vi "sortLinesAndVolumes.vi"(8 "error in (no error)":errorcluster, 9 "new volumes":T4(array[cluster]), 10 "Array of lines":T3(array[cluster]), 11 "assembler status":T2) -> (0 "error out":errorcluster, 1 "volumes to assemble":T1(array[cluster]), 2 "leftover lines":T3(array[cluster]), 3 "assembler status out":T2, 4 "num volume ends":i16, 5 "lines lost":i32)   [LabVIEW 2010]
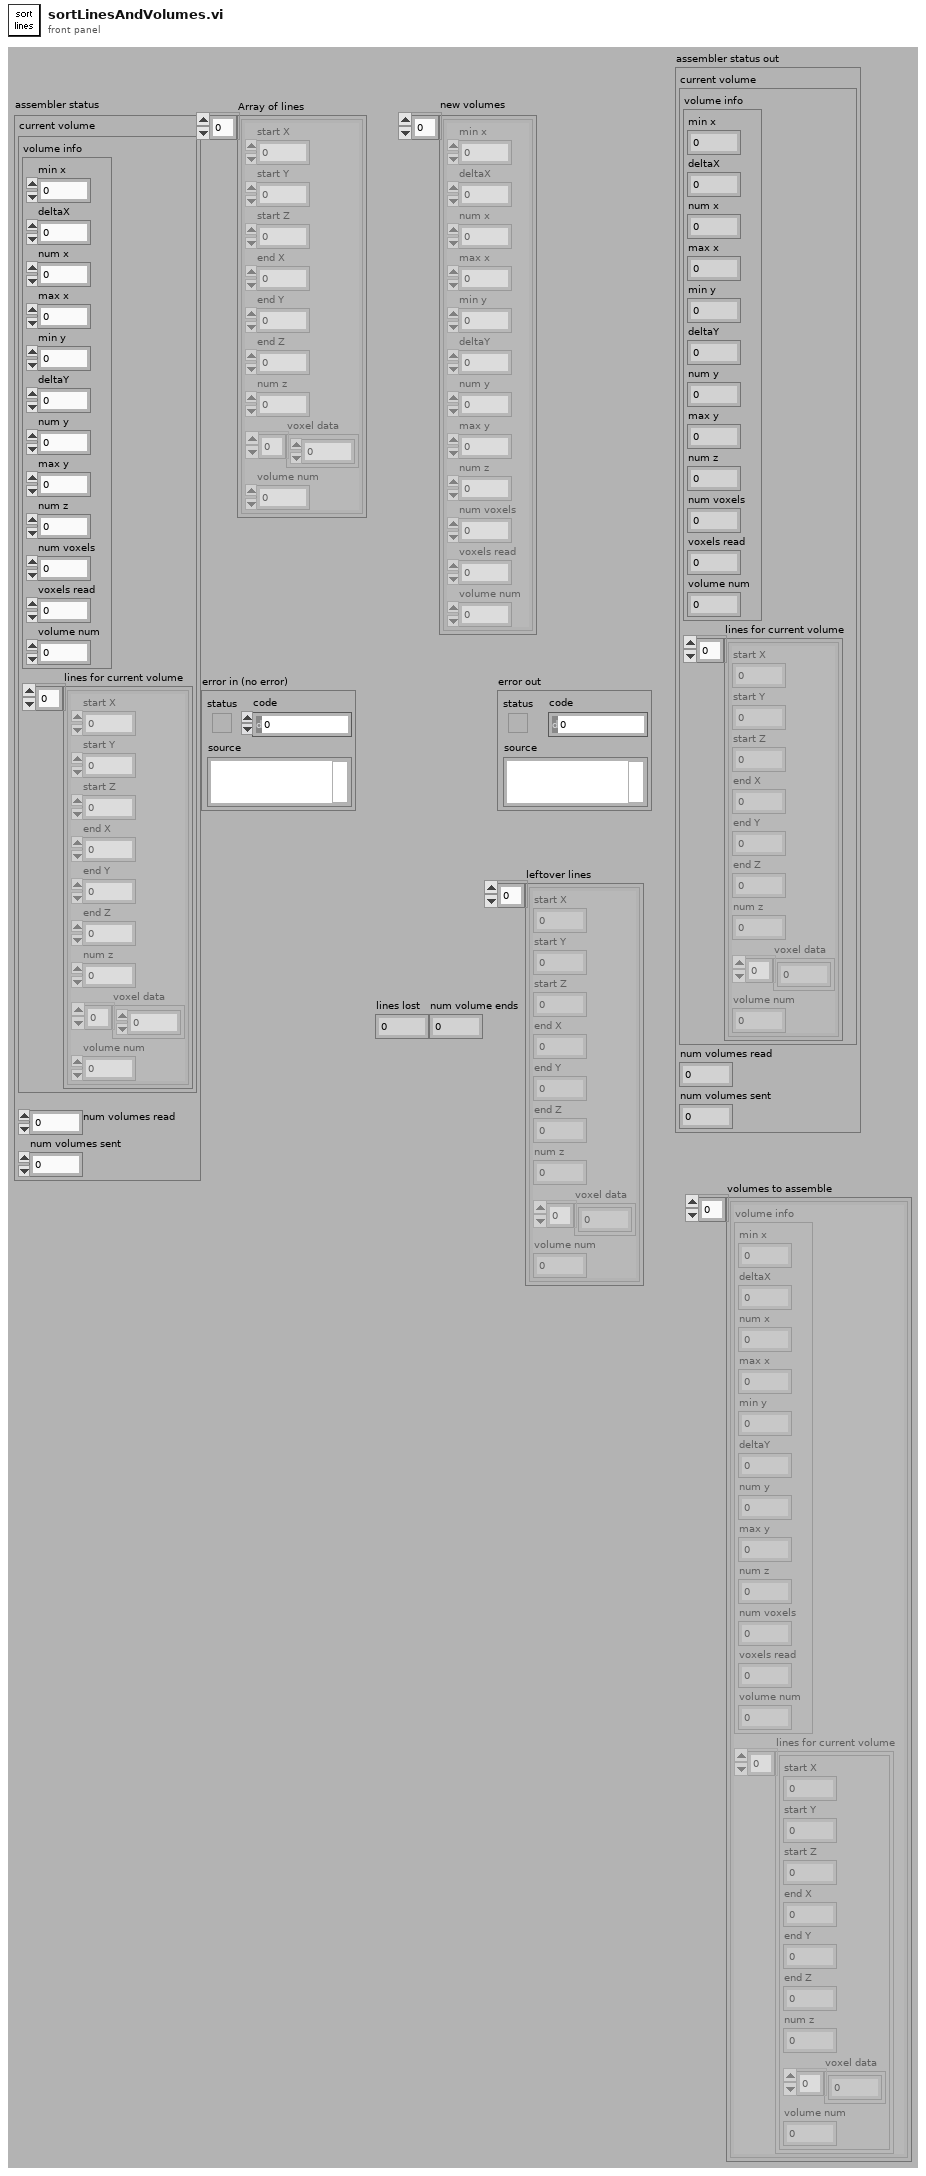
[diagram p1: front panel]
types:
  T1 = cluster{"volume info":cluster{"min x":i16, "deltaX":dbl, "num x":u32, "max x":i16, "min y":i16, "deltaY":dbl, "num y":u32, "max y":i16, "num z":u32, "num voxels":u32, "voxels read":u32, "volume num":u32}, "lines for current volume":cluster{"start X":i16, "start Y":i16, "start Z":i16, "end X":i16, "end Y":i16, "end Z":i16, "num z":u8, "voxel data":u32[], "volume num":u32}[]}[]
  T2 = cluster{"current volume":cluster{"volume info":cluster{"min x":i16, "deltaX":dbl, "num x":u32, "max x":i16, "min y":i16, "deltaY":dbl, "num y":u32, "max y":i16, "num z":u32, "num voxels":u32, "voxels read":u32, "volume num":u32}, "lines for current volume":cluster{"start X":i16, "start Y":i16, "start Z":i16, "end X":i16, "end Y":i16, "end Z":i16, "num z":u8, "voxel data":u32[], "volume num":u32}[]}, "num volumes read":u32, "num volumes sent":u32}
  T3 = cluster{"start X":i16, "start Y":i16, "start Z":i16, "end X":i16, "end Y":i16, "end Z":i16, "num z":u8, "voxel data":u32[], "volume num":u32}[]
  T4 = cluster{"min x":i16, "deltaX":dbl, "num x":u32, "max x":i16, "min y":i16, "deltaY":dbl, "num y":u32, "max y":i16, "num z":u32, "num voxels":u32, "voxels read":u32, "volume num":u32}[]
  T5 = cluster{"volume info":cluster{"min x":i16, "deltaX":dbl, "num x":u32, "max x":i16, "min y":i16, "deltaY":dbl, "num y":u32, "max y":i16, "num z":u32, "num voxels":u32, "voxels read":u32, "volume num":u32}, "lines for current volume":cluster{"start X":i16, "start Y":i16, "start Z":i16, "end X":i16, "end Y":i16, "end Z":i16, "num z":u8, "voxel data":u32[], "volume num":u32}[]}
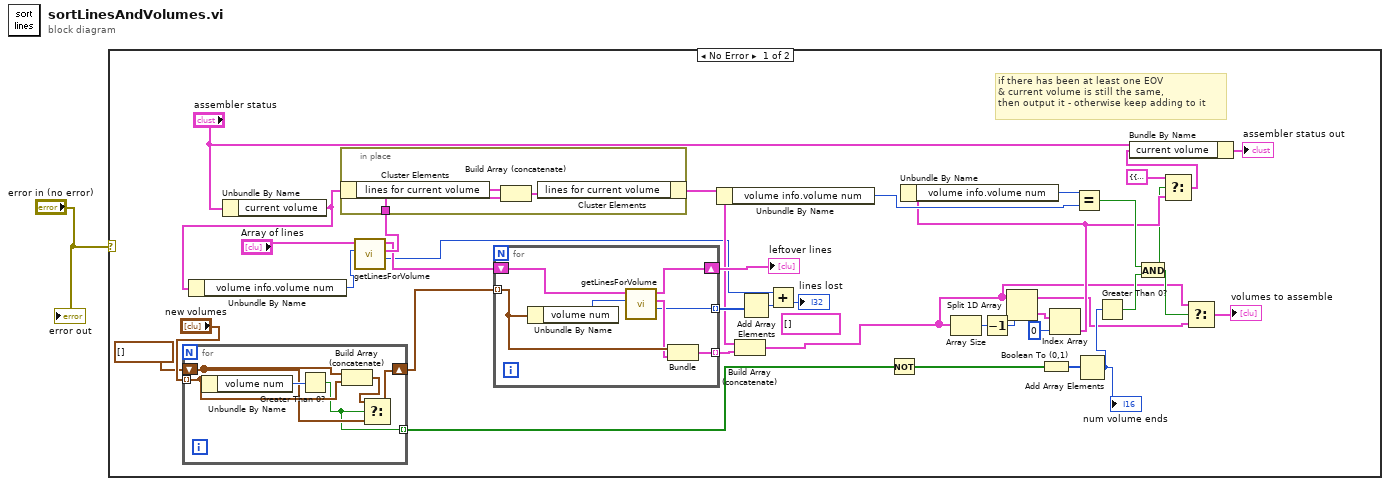
[diagram p0: block diagram]
diagram:
  n1 = case shown="No Error" "error in (no error)" {
    frame No Error {
      (unwired) T1 []
      # "if there has been at least one EOV\n& current volume is still the same,\nthen output it - otherwise keep adding to it"
      n2 = for {
        tunnel: "new volumes" -> [w42] mode=indexing
        shift-right: [w40] -> w5
        shift-left: T4 [] -> [w39]
        tunnel: [w38] -> w3 mode=indexing
        n3 = Unbundle By Name(w42) -> ("volume num"=w43:u32)
        n4 = Greater Than 0?(x=w43) -> (x > 0?=w38:bool)
        n5 = Build Array (concatenate)(w39, w42) -> (w41:T4)
        n6 = Select(t=w41, s=w38, f=w39) -> (s? t:f=w40:T4)
      }
      n7 = Unbundle By Name("assembler status") -> ("current volume"=w35:T5)
      n8 = Unbundle By Name(w35) -> ("volume info.volume num"=w36:u32)
      n9 = call "getLinesForVolume.vi"("volume num"=w36, "Array of lines"="Array of lines") -> ("lines lost"=w8:i32, "lines for current volume"=w34:T3, "lines for future volume"=w33:T3)  [unwired: 6 in, 1 out]
      n10 = in-place {
        in-place-border: w34 -> [w45]
        n11 = in-place-cluster #1(w35) -> ("lines for current volume"=w46:T3)
        n12 = Build Array (concatenate)(w46, w45) -> (w44:T3)
        n13 = in-place-cluster #1("lines for current volume"=w44) -> (w21:T5)
      }
      n14 = for {
        tunnel: w5 -> [w50] mode=indexing
        shift-right: [w52] -> w31
        shift-left: w33 -> [w53]
        tunnel: [w48] -> w32 mode=indexing
        tunnel: [w47] -> w28 mode=indexing
        n15 = Unbundle By Name(w50) -> ("volume num"=w51:u32)
        n16 = call "getLinesForVolume.vi"("volume num"=w51, "Array of lines"=w53) -> ("lines lost"=w48:i32, "lines for current volume"=w49:T3, "lines for future volume"=w52:T3)  [unwired: 6 in, 1 out]
        n17 = Bundle("volume info"=w50, "lines for current volume"=w49) -> (w47:T5)  [unwired: 1 in]
      }
      "leftover lines" <- w31
      n18 = Unbundle By Name(w21) -> ("volume info.volume num"=w19:u32)
      n19 = Build Array (concatenate)(w21, w28) -> (w2:T1)
      n20 = Add Array Elements(numeric array=w32) -> (sum=w30:i32)
      n21 = Add(x=w8, y=w30) -> (x+y=→"lines lost":i32)
      n22 = Not(x=w3) -> (.not. x?=w4:bool[])
      n23 = Array Size(array=w2) -> (size(s)=w25:i32)
      n24 = Decrement(x=w25) -> (x-1=w24:i32)
      n25 = Split 1D Array(array=w2, index=w24) -> (first subarray=w12:T1, second subarray=w23:T1)
      n26 = Boolean To (0,1)(Boolean=w4) -> (0, 1=w27:i16[])
      n27 = Index Array(array=w23, index=0) -> (element=w16:T5)
      n28 = Unbundle By Name(w16) -> ("volume info.volume num"=w20:u32)
      n29 = Equal?(x=w20, y=w19) -> (x = y?=w17:bool)
      n30 = Add Array Elements(numeric array=w27) -> (sum=w26:i16)
      "num volume ends" <- w26
      n31 = Greater Than 0?(x=w26) -> (x > 0?=w18:bool)
      n32 = And(x=w17, y=w18) -> (x .and. y?=w13:bool)
      n33 = Select(t=T5 {"volume info"={"min x"=0, "deltaX"=0.0, "num x"=0, "max x"=0, "min y"=0, "deltaY"=0.0, "num y"=0, "max y"=0, "num z"=0, "num voxels"=0, "voxels read"=0, "volume num"=0}, "lines for current volume"=[]}, s=w13, f=w16) -> (s? t:f=w14:T5)
      n34 = Bundle By Name(cluster="assembler status", "current volume"=w14) -> (→"assembler status out":T2)
      n35 = Select(t=w2, s=w13, f=w12) -> (s? t:f=→"volumes to assemble":T1)
    }
    frame Error {
    }
  }
  "error out" <- "error in (no error)"
